vi "Identificação MIMO (extended).vi"(6 "System Order":i32=4, 7 "Remove Trend":bool, 8 "Init Pump 2 voltage":dbl=3.0 min=0.0 format="%.2f", 9 "Init Pump 1 voltage":dbl=3.0 min=0.0 format="%.2f", 10 "Invert indentification and validation data?":bool, 11 "Stimulus and Response Signal":dbl[][](array[numeric])) -> (1 "output 2":dbl[][](graph) caption="Output H2", 2 "output 1":dbl[][](graph) caption="Output H1", 3 "Estimated MIMO State-space Model":picture, 5 "system model out":T1={"attributes"={"version"="1.0", "model type"=0, "input names"=[], "output names"=[], "notes"=""}, "coefficients"={"A "=[], "B"=[], "F"=[], "C"=[], "D"=[]}, "std deviations"={"A "=[], "B"=[], "F"=[], "C"=[], "D"=[]}, "coefficients covariance"=[], "noise variance"=[], "fs"=0.0, "system info"={"number of inputs"=0, "number of outputs"=0, "A order"=[], "B order"=[], "F order"=[], "C order"=[], "D order"=[], "Delays"=[]}, "kalman gain"=[], "initial state"=[], "trans func"=[], "zeros-poles"=[], "std of trans func"=[], "std of zeros-poles"=[], "trans func (noise)"=[], "std of trans func (noise)"=[], "zeros-poles (noise)"=[], "std of zeros-poles (noise)"=[], "Symbolic State Space Model"={"Symbolic A"=[], "Symbolic B"=[], "Symbolic C"=[], "Symbolic D"=[], "Symbolic K"=[], "Symbolic Initial State"=[]}, "delay"=[], "variables"=[], "grey trans func spec"={"orders of TF model"={" num order"=1, "den order"=2}, "# of zeros/poles at origin"={"zeros/poles"=1, "number "=0}, "delay initial?"=FALSE, "gain initial?"=FALSE}} {"grey trans func spec"."# of zeros/poles at origin"."zeros/poles" items=["zeros", "poles"]; "std of zeros-poles (noise)"."gain" format="%.2f"; "std of zeros-poles (noise)"."poles" format="%.2f"; "std of zeros-poles (noise)"."zeros" format="%.2f"; "zeros-poles (noise)"."gain" format="%.2f"; "zeros-poles (noise)"."poles" format="%.2f"; "zeros-poles (noise)"."zeros" format="%.2f"; "std of trans func (noise)"."alphas" format="%.2f"; "std of trans func (noise)"."betas" format="%.2f"; "trans func (noise)"."alphas" format="%.2f"; "trans func (noise)"."betas" format="%.2f"; "std of zeros-poles"."gain" format="%.2f"; "std of zeros-poles"."poles" format="%.2f"; "std of zeros-poles"."zeros" format="%.2f"; "std of trans func"."alphas" format="%.2f"; "std of trans func"."betas" format="%.2f"; "zeros-poles"."gain" format="%.2f"; "zeros-poles"."poles" format="%.2f"; "zeros-poles"."zeros" format="%.2f"; "trans func"."alphas" format="%.2f"; "trans func"."betas" format="%.2f"; "fs" format="%.2f"; "std deviations"."A" format="%.2f"; "std deviations"."D" format="%.2f"; "std deviations"."C" format="%.2f"; "std deviations"."F" format="%.2f"; "std deviations"."B" format="%.2f"; "coefficients"."A" format="%.2f"; "coefficients"."D" format="%.2f"; "coefficients"."C" format="%.2f"; "coefficients"."F" format="%.2f"; "coefficients"."B" format="%.2f"; "attributes"."model type" items=["Undefined", "AR", "ARX (SISO)", "ARX (MISO)", "ARX (MIMO)", "ARMAX (SISO)", "ARMAX (MISO)", "Output-Error (SISO)", "Output-Error (MISO)", "Box-Jenkins (SISO)", "Box-Jenkins (MISO)", "General Linear (SISO)", "General Linear (MISO)", "State-Space (SISO)", "State-Space (MISO)", "State-Space (MIMO)", "Transfer Function (SISO)", "Transfer Function (MISO)", "Transfer Function (MIMO)", "Zero-Pole-Gain (SISO)", "Zero-Pole-Gain (MISO)", "Zero-Pole-Gain (MIMO)"]})   [LabVIEW 2019]
uses:
  <vilib>/addons/System Identification/Model Typedefs.llb/si_generic model.ctl
  <vilib>/addons/System Identification/Model Typedefs.llb/SI Model Type.ctl
  <vilib>/addons/System Identification/Model Typedefs.llb/si_variables.ctl
  <vilib>/addons/System Identification/Data Preprocess.llb/SI Split Signal (MIMO Array).vi
  <vilib>/addons/System Identification/Data Preprocess.llb/SI Remove Trend (MIMO Array).vi
  GV Config.vi
  <vilib>/addons/System Identification/Parametric Estimation.llb/SI Estimate State-space Model (MIMO Array).vi
  <vilib>/addons/System Identification/Model Analysis.llb/SI Model Simulation (MIMO Array).vi
  <vilib>/addons/System Identification/NI_SysID.lvlib
panel:
  out "responses":dbl[][](array[numeric])
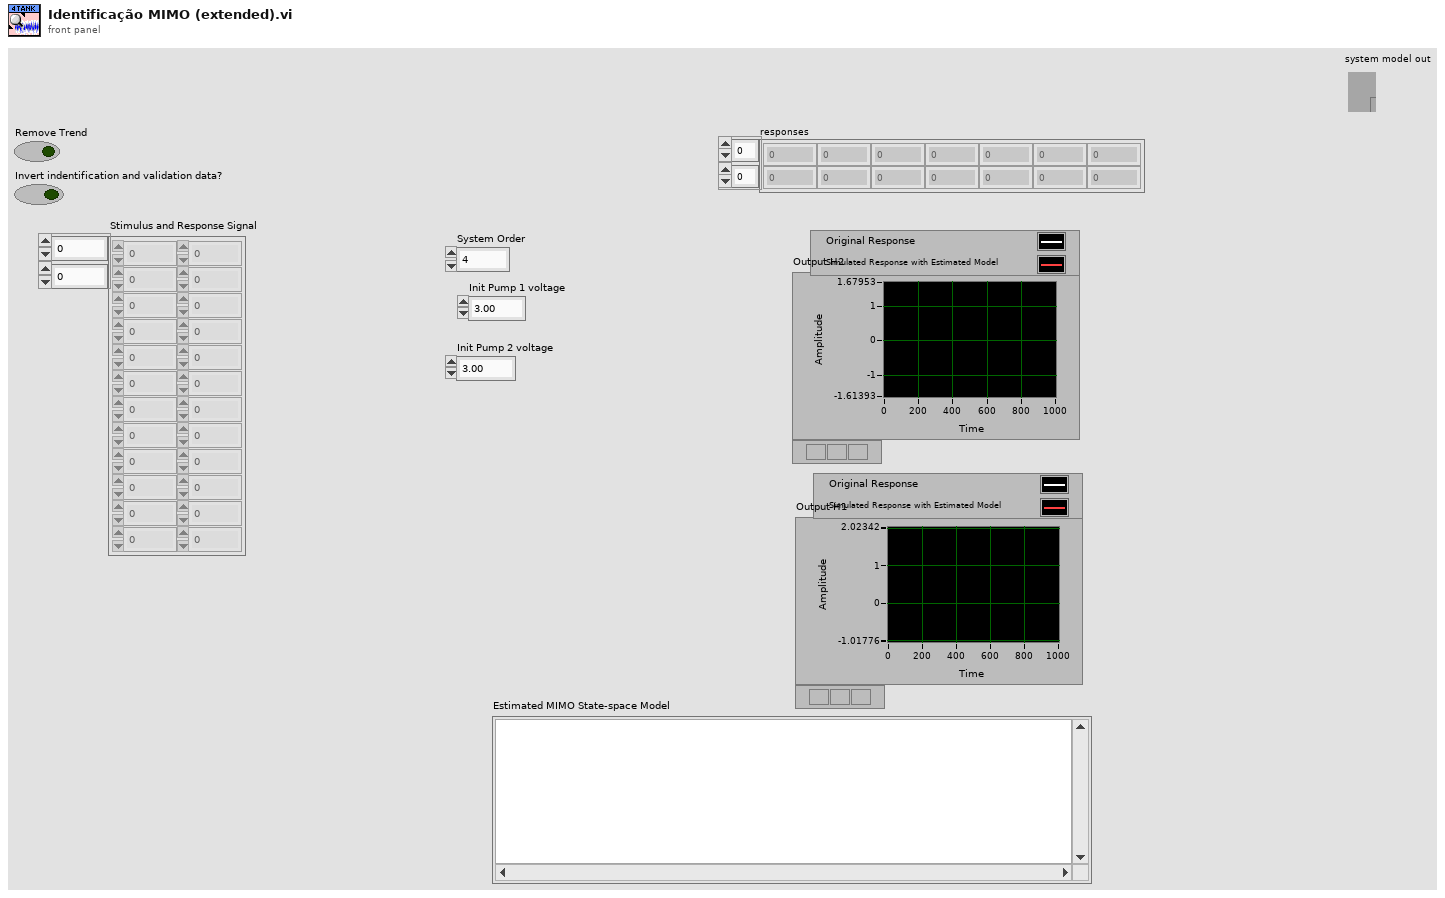
[diagram p1: front panel]
types:
  T1 = typedef "NI_SysID.lvlib/si_generic model.ctl" = cluster{"attributes":cluster{"version":string, "model type":T2, "input names":string[], "output names":string[], "notes":string}, "coefficients":cluster{"A ":dbl[][][], "B":dbl[][][], "F":dbl[][][], "C":dbl[][][], "D":dbl[][][]}, "std deviations":cluster{"A ":dbl[][][], "B":dbl[][][], "F":dbl[][][], "C":dbl[][][], "D":dbl[][][]}, "coefficients covariance":dbl[][][], "noise variance":dbl[][], "fs":dbl, "system info":cluster{"number of inputs":i32, "number of outputs":i32, "A order":i32[][], "B order":i32[][], "F order":i32[][], "C order":i32[][], "D order":i32[][], "Delays":i32[][]}, "kalman gain":dbl[][], "initial state":dbl[], "trans func":cluster{"betas":dbl[], "alphas":dbl[]}[][], "zeros-poles":cluster{"zeros":cdb[], "poles":cdb[], "gain":dbl}[][], "std of trans func":cluster{"betas":dbl[], "alphas":dbl[]}[][], "std of zeros-poles":cluster{"zeros":cdb[], "poles":cdb[], "gain":dbl}[][], "trans func (noise)":cluster{"betas":dbl[], "alphas":dbl[]}[][], "std of trans func (noise)":cluster{"betas":dbl[], "alphas":dbl[]}[][], "zeros-poles (noise)":cluster{"zeros":cdb[], "poles":cdb[], "gain":dbl}[][], "std of zeros-poles (noise)":cluster{"zeros":cdb[], "poles":cdb[], "gain":dbl}[][], "Symbolic State Space Model":cluster{"Symbolic A":string[][], "Symbolic B":string[][], "Symbolic C":string[][], "Symbolic D":string[][], "Symbolic K":string[][], "Symbolic Initial State":string[]}, "delay":dbl[][], "variables":T3, "grey trans func spec":cluster{"orders of TF model":cluster{" num order":i32, "den order":i32}, "# of zeros/poles at origin":cluster{"zeros/poles":u16, "number ":i32}, "delay initial?":bool, "gain initial?":bool}}
  T2 = typedef "NI_SysID.lvlib/SI Model Type.ctl" = u16
  T3 = typedef "NI_SysID.lvlib/si_variables.ctl" = cluster{"name":string, "initial guess":dbl, "upper limit":dbl, "lower limit":dbl, "value":dbl}[]
  T4 = cluster{"D matrix?":bool, "K matrix?":bool, "initial states?":bool}
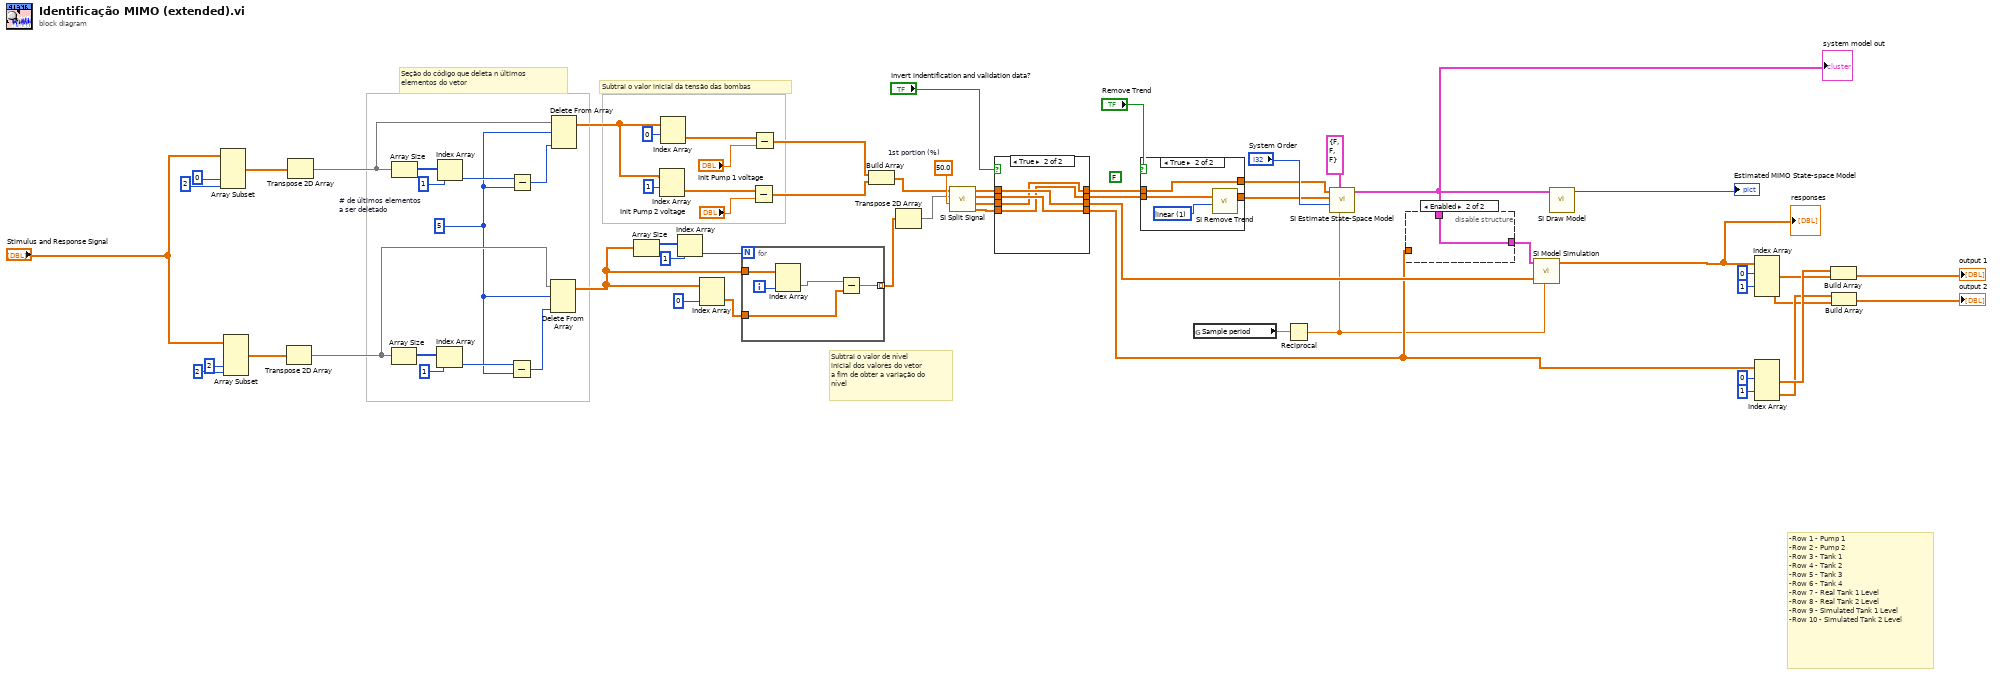
[diagram p0: block diagram]
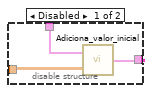
[diagram p4: hidden frame]
diagram:
  (unwired) FALSE
  w27 = 5  # # de últimos elementos  a ser deletado
  w60 = 50.0  # 1st portion (%)
  # "-Row 1 - Pump 1\n-Row 2 - Pump 2\n-Row 3 - Tank 1\n-Row 4 - Tank 2\n-Row 5 - Tank 3\n-Row 6 - Tank 4\n-Row 7 - Real Tank 1 Level\n-Row 8 - Real Tank 2 Level\n-Row 9 - Simulated Tank 1 Level\n-Row 10 - Simulated Tank 2 Level"
  # "Subtrai o valor inicial da tensão das bombas"
  # "Seção do código que deleta n últimos \nelementos do vetor"
  # "Subtrai o valor de nível \ninicial dos valores do vetor\na fim de obter a variação do\nnível"
  n1 = Array Subset(array="Stimulus and Response Signal", index (col)=0 ("index"), length (col)=2 ("length")) -> (w22:dbl[][])  [unwired: 2 in]
  n2 = Array Subset(array="Stimulus and Response Signal", index (col)=2 ("index"), length (col)=2 ("length")) -> (w21:dbl[][])  [unwired: 2 in]
  n3 = Transpose 2D Array(2D array=w21) -> (transposed array=w42:dbl[][])
  n4 = Transpose 2D Array(2D array=w22) -> (transposed array=w43:dbl[][])
  n5 = Array Size(array=w42) -> (size(s)=w58:i32[])
  n6 = Array Size(array=w43) -> (size(s)=w55:i32[])
  n7 = Index Array(array=w58, index=1) -> (element=w57:i32)
  n8 = Index Array(array=w55, index=1) -> (element=w56:i32)
  n9 = Subtract(x=w57, y=w27) -> (x-y=w39:i32)
  n10 = Subtract(x=w56, y=w27) -> (x-y=w38:i32)
  n11 = Delete From Array(array=w42, length=w27, index (col)=w39) -> (array with subset deleted=w33:dbl[][])  [unwired: 1 in, 1 out]
  n12 = Delete From Array(array=w43, length=w27, index (col)=w38) -> (array with subset deleted=w45:dbl[][])  [unwired: 1 in, 1 out]
  n13 = Array Size(array=w33) -> (size(s)=w32:i32[])
  n14 = Index Array(array=w45, index (row)=1 ("index")) -> (element=w53:dbl[])  [unwired: 1 in]
  n15 = Index Array(array=w45, index (row)=0 ("disabled index (col)")) -> (element=w54:dbl[])  [unwired: 1 in]
  n16 = Index Array(array=w32, index=1) -> (element=w30:i32)
  n17 = Index Array(array=w33, index (col)=0 ("index (row)")) -> (element=w59:dbl[])  [unwired: 1 in]
  n18 = for {
    N: w30 -> [_]
    tunnel: w59 -> [w72]
    tunnel: w33 -> [w70]
    tunnel: [w71] -> w28 mode=indexing
    i -> [w69]
    n19 = Index Array(array=w70, index (col)=w69) -> (element=w68:dbl[])  [unwired: 1 in]
    n20 = Subtract(x=w68, y=w72) -> (x-y=w71:dbl[])
  }
  n21 = Subtract(x=w53, y="Init Pump 2 voltage") -> (x-y=w52:dbl[])
  n22 = Subtract(x=w54, y="Init Pump 1 voltage") -> (x-y=w44:dbl[])
  n23 = Build Array(w44, w52) -> (w35:dbl[][])
  n24 = Transpose 2D Array(2D array=w28) -> (transposed array=w29:dbl[][])
  n25 = call-poly <vilib>:"SI Split Signal.vi"("1st portion (%)"=w60, "response signals in"=w29, "stimulus signals in"=w35) -> ("response signals 2"=w3:dbl[][], "stimulus signals 2"=w5:dbl[][], "response signals 1"=w7:dbl[][], "stimulus signals 1"=w9:dbl[][])  [unwired: 5 in]
  n26 = case shown="True" "Invert indentification and validation data?" {
    tunnel: [w76 w78] -> w10
    tunnel: w9 -> [w76 w80]
    tunnel: [w75 w77] -> w8
    tunnel: w7 -> [w75 w79]
    tunnel: [w74 w80] -> w6
    tunnel: w5 -> [w74 w78]
    tunnel: [w73 w79] -> w4
    tunnel: w3 -> [w73 w77]
    frame False {
    }
    frame True {
    }
  }
  n27 = case shown="True" "Remove Trend" {
    tunnel: w10 -> [w81 w83]
    tunnel: w8 -> [w82 w86]
    tunnel: [w82 w85] -> w16
    tunnel: [w81 w83] -> w14
    frame False {
    }
    frame True {
      w84 = 1 items=["mean", "linear"] ("trend type")
      n28 = call-poly <vilib>:"SI Remove Trend.vi"("trend type"=w84, "response signals in"=w86) -> ("response signals out"=w85:dbl[][])  [unwired: 5 in, 4 out]
    }
  }
  n29 = global read "GV Config.vi" "Sample period"() -> (w2:dbl)
  n30 = Reciprocal(x=w2) -> (1/x=w1:dbl)
  n31 = call-poly <vilib>:"SI Estimate State-Space Model.vi"("sampling rate (Hz)"=w1, "structure selector"=T4 {"D matrix?"=FALSE, "K matrix?"=FALSE, "initial states?"=FALSE}, "number of states"="System Order", "response signals"=w16, "stimulus signals"=w14) -> ("system model out"=w13:T1)  [unwired: 1 in, 5 out]
  "system model out" <- w13
  n32 = disable-structure shown="Enabled" {
    disable-tunnel: w4 -> [w88 _]
    disable-tunnel: [w87 w90] -> w12
    disable-tunnel: w13 -> [w89 w90]
    frame Disabled {
      n33 = call "Adiciona_valor_inicial.vi"("Array"=w88, "system model in"=w89) -> ("system model out"=w87:T1)
    }
    frame Enabled {
    }
  }
  n34 = call-poly <vilib>:"SI Model Simulation.vi"("sampling rate (Hz)"=w1, "stimulus signals"=w6, "system model"=w12) -> ("responses"=w19:dbl[][])  [unwired: 6 in, 2 out]
  "responses" <- w19
  n35 = call <vilib>:"SI Draw Model.vi"("system model"=w13) -> ("model"=→"Estimated MIMO State-space Model":picture)  [unwired: 8 in, 2 out]
  n36 = Index Array(array=w19, index (row) #1=0 ("disabled index (col)"), index (row) #2=1 ("index (col)")) -> (element #1=w47:dbl[], element #2=w46:dbl[])  [unwired: 2 in]
  n37 = Index Array(array=w4, index (row) #1=0 ("disabled index (col)"), index (row) #2=1 ("index (col)")) -> (element #1=w49:dbl[], element #2=w48:dbl[])  [unwired: 2 in]
  n38 = Build Array(w49, w47) -> (→"output 1":dbl[][])
  n39 = Build Array(w48, w46) -> (→"output 2":dbl[][])
